vi "Configure Control Mode.vi"(8 "error in (no error)":errorcluster, 9 "Control Mode (0:ATTenuation)":u16(ring) items=["ATTenuation", "POWer"], 10 "Platform Slot Number (10)":i16=10 min=-1 max=255, 11 "VISA resource name":refnum<visa-resource-name>) -> (0 "error out":errorcluster, 3 "VISA resource name out":refnum<visa-resource-name>)   [LabVIEW 2018, in "LTB-1.lvlib" / "3150.lvlib"]
doc: "Configures the attenuator's control mode."
uses:
  3150.lvlib
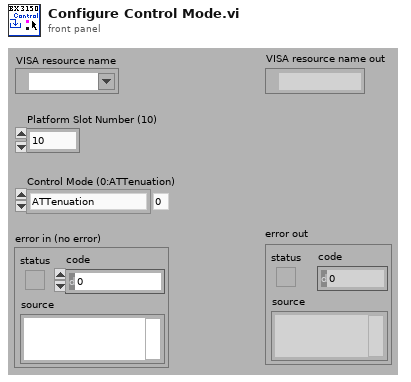
[diagram p1: front panel]
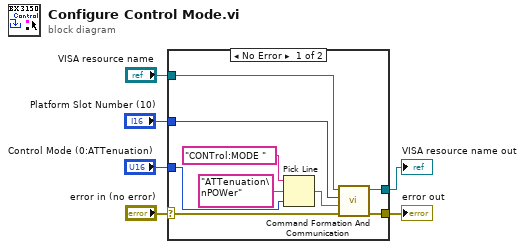
[diagram p0: block diagram]
diagram:
  n1 = case shown="No Error" "error in (no error)" {
    selector: "error in (no error)" -> [w14 w16]
    tunnel: "VISA resource name" -> [w15 w17]
    tunnel: [w13 w17] -> w4
    tunnel: [w12 w16] -> w3
    tunnel: "Control Mode (0:ATTenuation)" -> [w10 _]
    tunnel: "Platform Slot Number (10)" -> [w7 _]
    frame No Error {
      n2 = Pick Line(string ("")="CONTrol:MODE " ("Command"), multi-line string="ATTenuation\nPOWer", line index=w10) -> (output string=w8:string)
      n3 = call "Command Formation And Communication.vi"("error in (no error)"=w14, "Command"=w8, "Platform Slot Number"=w7, "VISA resource name"=w15) -> ("error out"=w12:errorcluster, "VISA resource name out"=w13:refnum<visa-resource-name>)  [unwired: 1 in, 5 out]
    }
    frame Error {
    }
  }
  "VISA resource name out" <- w4
  "error out" <- w3
